vi "8164B ReadNLineResponse.vi"(8 "error in":errorcluster, 10 "Number of lines to read":i32, 11 "KeySight 8164B control in":T1) -> (0 "error out":errorcluster, 2 "NLineResponse":string[](array[string]), 3 "KeySight 8164B control out":T1)   [LabVIEW 2018, in "KeySight 8164B LAN InstrLib.lvlib"]
uses:
  KeySight 8164B LAN InstrLib.lvlib
  typedefs/KeySight 8164B control.ctl
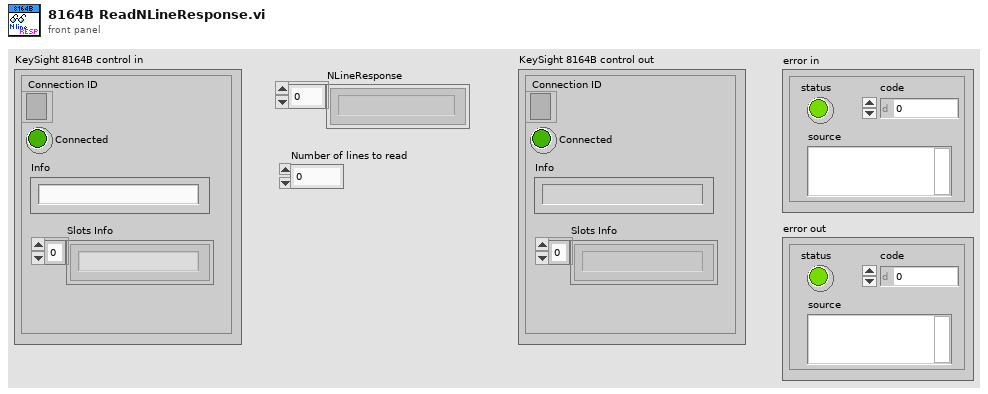
[diagram p1: front panel]
types:
  T1 = typedef "KeySight 8164B LAN InstrLib.lvlib/KeySight 8164B control.ctl" = cluster{"Connection ID":refnum<k5>, "Connected":bool, "Info":string, "Slots Info":string[]}
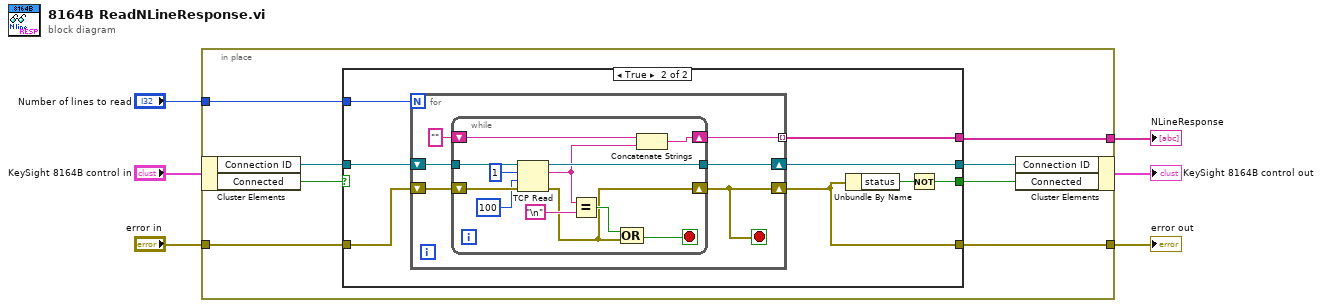
[diagram p0: block diagram]
diagram:
  n1 = in-place {
    in-place-border: "error in" -> [w12]
    in-place-border: [w11] -> w3
    in-place-border: [w10] -> w2
    in-place-border: "Number of lines to read" -> [w7]
    n2 = in-place-cluster #1("KeySight 8164B control in") -> ("Connection ID"=w13:refnum<k5>, "Connected"=w9:bool)
    n3 = case shown="True" w9 {
      selector: w9 -> [w16 _]
      tunnel: [w17 w25] -> w14
      tunnel: w13 -> [w17 w24]
      tunnel: w12 -> [w15 w23]
      tunnel: [w15 w22] -> w11
      tunnel: [_ w19] -> w10
      tunnel: [w16 w20] -> w8
      tunnel: w7 -> [_ w18]
      frame False {
      }
      frame True {
        n4 = for {
          N: w18 -> [_]
          shift-right: [w31] -> w25
          shift-left: w24 -> [w30]
          shift-right: [w26] -> w22
          shift-left: w23 -> [w29]
          tunnel: [w27] -> w19 mode=indexing
          stop <- w26 stop-if-true
          n5 = while {
            tunnel: w30 -> [w43]
            tunnel: [w37] -> w31
            shift-right: [w36] -> w26
            shift-left: w29 -> [w41]
            shift-right: [w33] -> w27
            shift-left: "" -> [w35]
            stop <- w40 stop-if-true
            n6 = TCP Read(connection ID=w43, bytes to read=1, error in (no error)=w41, 9:100 ("timeout ms (25000)")) -> (connection ID out=w37:refnum<k5>, data out=w34:string, error out=w36:errorcluster)  [unwired: 1 in]
            n7 = Equal?(x=w34, y="\n") -> (x = y?=w38:bool)
            n8 = Compound Arithmetic op=OR(w38, w36) -> (w40:bool)
            n9 = Concatenate Strings(w35, w34) -> (w33:string)
          }
        }
        n10 = Unbundle By Name(w22) -> ("status"=w21:bool)
        n11 = Not(x=w21) -> (.not. x?=w20:bool)
      }
    }
    n12 = in-place-cluster #1("Connection ID"=w14, "Connected"=w8) -> (→"KeySight 8164B control out":T1)
  }
  "error out" <- w3
  "NLineResponse" <- w2
